vi "Host - Initialise and clone (SubVI).vi"(7 "Pilot":bool, 8 "error in":errorcluster, 10 "Tab Reference":refnum<vi>) -> (0 "error out":errorcluster, 2 "Control names":string[](array[string]), 3 "Data Cluster":T2={"VI References"=[], "Addresses"=[], "Pilot"=FALSE, "DO Data"=[], "Access Restricted?"=FALSE, "Pilot Control References"=[], "CoPilot Control References"=[], "cRIO Config"=[], "datalog Q"=refnum, "PS_P"={"AI"=[], "DI"=[], "DO"=[], "Serial"=[], "CPU"={"Total Load"=[], "Interrupt Load"=[], "Total Physical"=0.0, "Free Physical"=0.0, "Primary Disk Capacity"=0.0, "Primary Disk Free"=0.0}, "Stop"=FALSE, "DO Channel"=[]}, "PS_S"={"AI"=[], "DI"=[], "DO"=[], "Serial"=[], "CPU"={"Total Load"=[], "Interrupt Load"=[], "Total Physical"=0.0, "Free Physical"=0.0, "Primary Disk Capacity"=0.0, "Primary Disk Free"=0.0}, "Stop"=FALSE, "DO Channel"=[]}, "IDE_P"={"AI"=[], "DI"=[], "DO"=[], "Serial"=[], "CPU"={"Total Load"=[], "Interrupt Load"=[], "Total Physical"=0.0, "Free Physical"=0.0, "Primary Disk Capacity"=0.0, "Primary Disk Free"=0.0}, "Stop"=FALSE, "DO Channel"=[]}, "IDE_S"={"AI"=[], "DI"=[], "DO"=[], "Serial"=[], "CPU"={"Total Load"=[], "Interrupt Load"=[], "Total Physical"=0.0, "Free Physical"=0.0, "Primary Disk Capacity"=0.0, "Primary Disk Free"=0.0}, "Stop"=FALSE, "DO Channel"=[]}, "PDE_P"={"AI"=[], "DI"=[], "DO"=[], "Serial"=[], "CPU"={"Total Load"=[], "Interrupt Load"=[], "Total Physical"=0.0, "Free Physical"=0.0, "Primary Disk Capacity"=0.0, "Primary Disk Free"=0.0}, "Stop"=FALSE, "DO Channel"=[]}, "PDE_S"={"AI"=[], "DI"=[], "DO"=[], "Serial"=[], "CPU"={"Total Load"=[], "Interrupt Load"=[], "Total Physical"=0.0, "Free Physical"=0.0, "Primary Disk Capacity"=0.0, "Primary Disk Free"=0.0}, "Stop"=FALSE, "DO Channel"=[]}, "GUI References"={"Control Names"=[], "Control References"=[]}, "GUI Data"=[], "TCP - Serial"=[], "TCP-Serial Q"=refnum, "TCP Serial Ref"=[], "Data Sets"=[], "Last Data"=[], "Alarm Data"=[], "DI Data"=[], "Ack Data"=[], "Buzzer Data"=[], "Pilot DO"=[], "Co-Pilot DO"=[], "System Down?"=FALSE, "Log Data"=[], "Update Array"=[], "MCC Data Log"=[], "MCC Data Not"=refnum, "Thruster control"=[refnum, refnum, refnum, refnum, refnum, refnum, refnum, refnum, refnum], "waga notifier out"=refnum, "Wago  log"=[], "Thruster Cont"=[0.0, 0.0, 0.0, 0.0, 0.0, 0.0, 0.0, 0.0, 0.0], "Cam Cont"=[FALSE, FALSE, FALSE, FALSE, FALSE, TRUE], "PDE_P TH Cont"={"COM 10"=0.0, "COM 11"=0.0, "COM 12"=0.0, "COM 13"=0.0}, "PDE_S TH Cont"={"COM 10"=0.0, "COM 11"=0.0, "COM 12"=0.0, "COM 13"=0.0}} {"cRIO Config"."AI"."Interface Data"."Timing"."sample mode" items=["Finite Samples"=10178, "Continuous Samples"=10123, "Hardware Timed Single Point"=12522]; "cRIO Config"."Async"."Interface Data"."Data"."Minor Frame Count" min=5 max=8 step=1})   [LabVIEW 2021]
uses:
  Analog Output/Controls/AO Channel Configuration Cluster.ctl
  Analog Output/Controls/AO Timing Cluster.ctl
  Analog Output/Controls/AO Interface Data Cluster.ctl
  Analog Output/Controls/AO JSON Data Cluster.ctl
  Digital Output/SubVIs/Digital Dynamic Cluster.ctl
  Digital Output/Controls/DIO Interface Data.ctl
  Digital Output/Controls/DIO Configuration cluster.ctl
  Async Serial/Controls/Async Message Info Cluster.ctl
  Async Serial/Controls/Async Frame Info Cluster.ctl
  Async Serial/Controls/Async Serial Configuration Cluster.ctl
  Async Interface Data Cluster.ctl
  Async JSON Cluster.ctl
  Main Engine/Controls/Main Engine CPU Info.ctl
  Controls/Host Data Cluster.ctl
  Controls/Host - GUI Data Cluster.ctl
  Async Serial/Controls/Async Sensor Type.ctl
panel:
  out "Array":u32[](array[numeric])
  out "output array":refnum<vi>[](array[refnum])
  out "Names 3":string[](array[string])
  out "Names":string[](array[string])
  in  "Sensor Type":T1=enum."INS"
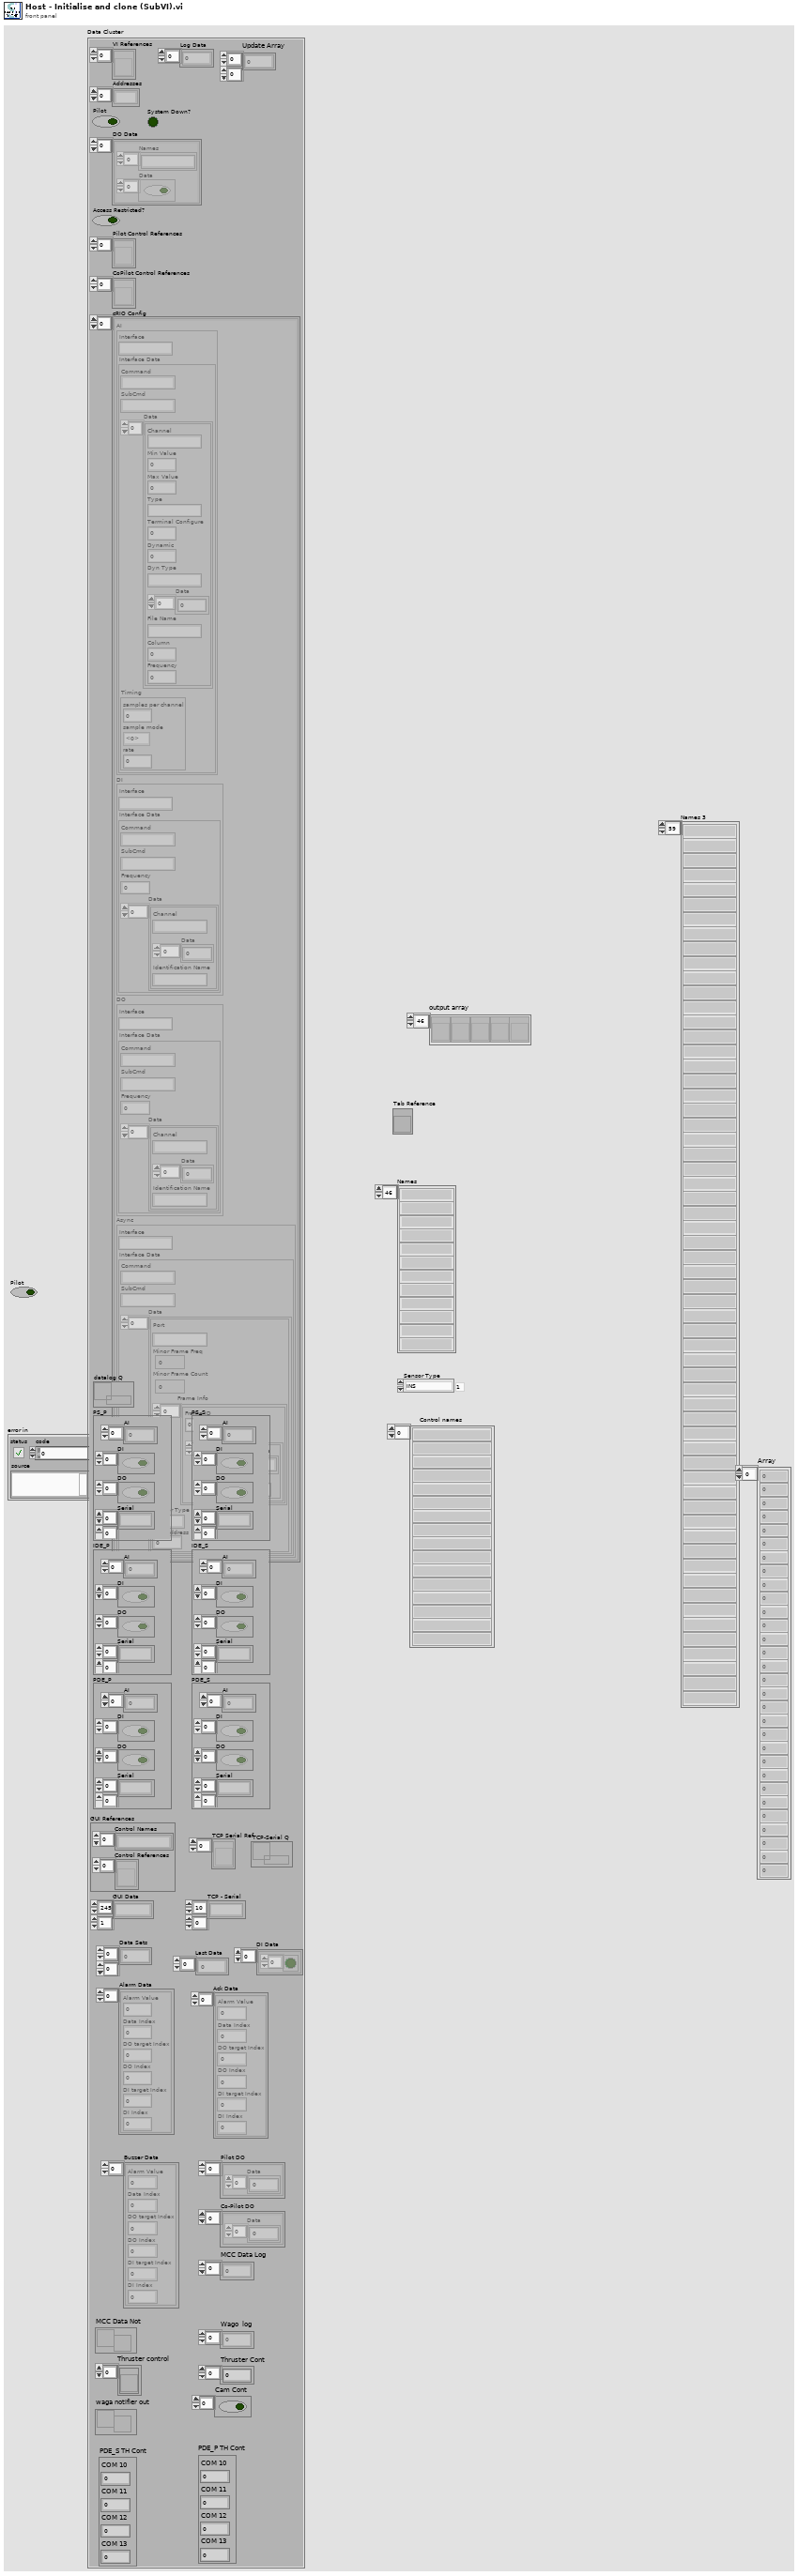
[diagram p1: front panel]
types:
  T1 = typedef "Async Sensor Type.ctl" = enum16{"Camera", "INS", "Pri BMS", "Aux BMS", "Depth Sensor", "Altimeter", "OIM", "Thruster", "Acoustic Modem", "LED"}
  T2 = typedef "Host - GUI Data Cluster.ctl" = cluster{"VI References":refnum<vi>[], "Addresses":string[], "Pilot":bool, "DO Data":cluster{"Names":string[], "Data":bool[]}[], "Access Restricted?":bool, "Pilot Control References":refnum<vi>[], "CoPilot Control References":refnum<vi>[], "cRIO Config":cluster{"AI":T3, "DI":T7, "DO":T7, "Async":T10}[], "datalog Q":refnum<queue>, "PS_P":T15, "PS_S":T15, "IDE_P":T15, "IDE_S":T15, "PDE_P":T15, "PDE_S":T15, "GUI References":cluster{"Control Names":string[], "Control References":refnum<vi>[]}, "GUI Data":string[][], "TCP - Serial":string[][], "TCP-Serial Q":refnum<queue>, "TCP Serial Ref":refnum<vi>[], "Data Sets":dbl[][], "Last Data":dbl[], "Alarm Data":cluster{"Alarm Value":dbl, "Data Index":i32, "DO target Index":i32, "DO Index":i32, "DI target Index":i32, "DI Index":i32}[], "DI Data":cluster{bool[]}[], "Ack Data":cluster{"Alarm Value":dbl, "Data Index":i32, "DO target Index":i32, "DO Index":i32, "DI target Index":i32, "DI Index":i32}[], "Buzzer Data":cluster{"Alarm Value":dbl, "Data Index":i32, "DO target Index":i32, "DO Index":i32, "DI target Index":i32, "DI Index":i32}[], "Pilot DO":cluster{"Data":i32[]}[], "Co-Pilot DO":cluster{"Data":i32[]}[], "System Down?":bool, "Log Data":dbl[], "Update Array":i32[][], "MCC Data Log":dbl[], "MCC Data Not":refnum<notifier>, "Thruster control":refnum<vi>[], "waga notifier out":refnum<notifier>, "Wago  log":sgl[], "Thruster Cont":dbl[], "Cam Cont":bool[], "PDE_P TH Cont":cluster{"COM 10":dbl, "COM 11":dbl, "COM 12":dbl, "COM 13":dbl}, "PDE_S TH Cont":cluster{"COM 10":dbl, "COM 11":dbl, "COM 12":dbl, "COM 13":dbl}}
  T3 = typedef "AO JSON Data Cluster.ctl" = cluster{"Interface":string, "Interface Data":T4}
  T4 = typedef "AO Interface Data Cluster.ctl" = cluster{"Command":string, "SubCmd":string, "Data":T5[], "Timing":T6}
  T5 = typedef "AO Channel Configuration Cluster.ctl" = cluster{"Channel":string, "Min Value":dbl, "Max Value":dbl, "Type":string, "Terminal Configure":u16, "Dynamic":u8, "Dyn Type":string, "Data":dbl[], "File Name":string, "Column":i32, "Frequency":dbl}
  T6 = typedef "AO Timing Cluster.ctl" = cluster{"samples per channel":i32, "sample mode":i32, "rate":dbl}
  T7 = typedef "DIO Configuration cluster.ctl" = cluster{"Interface":string, "Interface Data":T8}
  T8 = typedef "DIO Interface Data.ctl" = cluster{"Command":string, "SubCmd":string, "Frequency":u16, "Data":T9[]}
  T9 = typedef "Digital Dynamic Cluster.ctl" = cluster{"Channel":string, "Data":u8[], "Identification Name":string}
  T10 = typedef "Async JSON Cluster.ctl" = cluster{"Interface":string, "Interface Data":T11}
  T11 = typedef "Async Interface Data Cluster.ctl" = cluster{"Command":string, "SubCmd":string, "Data":T12[]}
  T12 = typedef "Async Serial Configuration Cluster.ctl" = cluster{"Port":string, "Minor Frame Freq":u16, "Minor Frame Count":u16, "Frame Info":T13[], "Sensor Type":u16, "OIM Address":u16}
  T13 = typedef "Async Frame Info Cluster.ctl" = cluster{"Frame ID":u16, "Message Info":T14[]}
  T14 = typedef "Async Message Info Cluster.ctl" = cluster{"Message":u8[], "Message Name":string}
  T15 = typedef "Host Data Cluster.ctl" = cluster{"AI":dbl[], "DI":bool[], "DO":bool[], "Serial":string[][], "CPU":T16, "Stop":bool, "DO Channel":string[]}
  T16 = typedef "Main Engine CPU Info.ctl" = cluster{"Total Load":u32[], "Interrupt Load":u32[], "Total Physical":dbl, "Free Physical":dbl, "Primary Disk Capacity":dbl, "Primary Disk Free":dbl}
  T17 = cluster{"AI":T3, "DI":T7, "DO":T7, "Async":T10}[]
  T18 = cluster{"Alarm Value":dbl, "Data Index":i32, "DO target Index":i32, "DO Index":i32, "DI target Index":i32, "DI Index":i32}[]
diagram:
  (unwired) string[][] [["IDE_P Voltage (V)", "IDE_P/AI/0", "3", "20", "PS_S/DO/0", "PS_S/DI/0", "0", "40", "25"], ["IDE_P_Voltage_2", "IDE_P/AI/1", "", "", "", "", "1", "-1", "-1"], ["IDE_P_Temp", "IDE_P/AI/2", "", "", "", "", "2", "-1", "27"], ["IDE_P Current (A)", "IDE_P/AI/3", ".05", "", "", "", "3", "41", "26"], ["IDE_P_Current_2", "IDE_P/AI/4", "", "", "", "", "4", "-1", "-1"], ["IDE_P WIS 1", "IDE_P/AI/5", "", "", "", "", "6", "-1", "-1"], ["IDE_P WIS 2", "IDE_P/AI/6", "", "", "", "", "7", "-1", "-1"], ["IDE_S Voltage (V)", "IDE_S/AI/0", "3", "", "", "", "8", "28", "20"], ["IDE_S_Voltage_2", "IDE_S/AI/1", "", "", "", "", "9", "-1", "-1"], ["IDE_S_Temp", "IDE_S/AI/2", "", "", "", "", "10", "-1", "22"], ["IDE_S Current (A)", "IDE_S/AI/3", "5", "", "", "", "11", "29", "21"], ["IDE_S_Current_2", "IDE_S/AI/4", "", "", "", "", "12", "-1", "-1"], ["IDE_S WIS 1", "IDE_S/AI/5", "", "", "", "", "14", "-1", "-1"], ["IDE_S WIS 2", "IDE_S/AI/6", "", "", "", "", "15", "-1", "-1"], ["PDE_P Voltage (V)", "PDE_P/AI/0", "16", "", "", "", "16", "38", "35"], ["PDE_P Current (A)", "PDE_P/AI/1", "30", "", "", "", "17", "39", "36"], ["PDE_P 24 Voltage1 (V)", "PDE_P/AI/2", "", "", "", "", "18", "-1", ""], ["PDE_P 24Current (A)", "PDE_P/AI/3", "", "", "", "", "19", "-1", ""], ["PDE_P 24 Voltage2 (V)", "PDE_P/AI/4", "", "", "", "", "20", "-1", ""], ["T1 Current", "PDE_P/AI/5", "7.5", "", "", "", "21", "-1", ""], ["T3 Current", "PDE_P/AI/6", "7.5", "", "", "", "22", "-1", ""], ["T5 Current", "PDE_P/AI/7", "7.5", "", "", "", "23", "-1", ""], ["T7 Current", "PDE_P/AI/8", "7.5", "", "", "", "24", "-1", ""], ["PDE_P BATS CUR", "PDE_P/AI/9", "", "", "", "", "25", "-1", ""], ["", "PDE_P/AI/10", "", "", "", "", "-1", "-1", ""], ["PDE_P Temp (degC)", "PDE_P/AI/12", "", "", "", "", "28", "-1", "37"], ["PDE_S Voltage (V)", "PDE_S/AI/0", "20", "", "", "", "29", "26", "30"], ["PDE_S Current (A)", "PDE_S/AI/1", "30", "", "", "", "30", "27", "31"], ["PDE_S24VOL1", "PDE_S/AI/2", "", "", "", "", "31", "-1", ""], ["PDE_S24V CUR", "PDE_S/AI/3", "", "", "", "", "32", "-1", ""], ["PDE_S24VOL2", "PDE_S/AI/4", "", "", "", "", "33", "-1", ""], ["T2 Current", "PDE_S/AI/5", "7.5", "", "", "", "34", "-1", ""], ["T4 Current", "PDE_S/AI/6", "7.5", "", "", "", "35", "-1", ""], ["T6 Current", "PDE_S/AI/7", "7.5", "", "", "", "36", "-1", ""], ["T8 Current", "PDE_S/AI/8", "7.5", "", "", "", "37", "-1", ""], ["PDE_S BATS CUR", "PDE_S/AI/9", "", "", "", "", "38", "-1", ""], ["LS01", "PDE_S/AI/10", "", "", "", "", "-1", "-1", ""], ["PDE_S_Temp", "PDE_S/AI/11", "", "", "", "", "41", "-1", "32"], ["4K camera P", "IDE_P/DO/0", "", "", "", "", "-1", "-1", ""], ["HD Camera P1", "IDE_P/DO/1", "", "", "", "", "-1", "-1", ""], ["HD Camera P2", "IDE_P/DO/2", "", "", "", "", "-1", "-1", ""], ["HD Camera P3", "IDE_P/DO/3", "", "", "", "", "-1", "-1", ""], ["SD_Camera_P4", "IDE_P/DO/4", "", "", "", "", "-1", "-1", ""], ["Pan and Tilt P1", "IDE_P/DO/5", "", "", "", "", "-1", "-1", ""], ["Laser Light 2", "IDE_P/DO/6", "", "", "", "", "-1", "-1", ""], ["LED Light P2", "IDE_P/DO/7", "", "", "", "", "-1", "-1", ""], ["LED Light P3", "IDE_P/DO/8", "", "", "", "", "-1", "-1", ""], ["LED Light P4", "IDE_P/DO/9", "", "", "", "", "-1", "-1", ""], ["Pan and Tilt P2", "IDE_P/DO/10", "", "", "", "", "-1", "-1", ""], ["Laser Light 1", "IDE_P/DO/11", "", "", "", "", "-1", "-1", ""], ["Depth Sensor Pri", "IDE_P/DO/12", "", "", "", "", "-1", "-1", ""], ["INS-DVL", "IDE_P/DO/13", "", "", "", "", "-1", "-1", ""], ["Multibeam Sonar", "IDE_P/DO/39", "", "", "", "", "-1", "-1", ""], ["SVP, Turbidity, pH", "IDE_P/DO/33", "", "", "", "", "-1", "-1", ""], ["CO2 Sensor", "IDE_P/DO/34", "", "", "", "", "-1", "-1", ""], ["Trim System", "IDE_P/DO/35", "", "", "", "", "-1", "-1", ""], ["Methane_Sensor", "IDE_P/DO/36", "", "", "", "", "-1", "-1", ""], ["VBS", "IDE_P/DO/37", "", "", "", "", "-1", "-1", ""], ["MBS", "IDE_P/DO/39", "", "", "", "", "-1", "-1", ""], ["4K camera S", "IDE_S/DO/0", "", "", "", "", "-1", "-1", ""], ["HD Camera S1", "IDE_S/DO/1", "", "", "", "", "-1", "-1", ""], ["HD Camera S2", "IDE_S/DO/2", "", "", "", "", "-1", "-1", ""], ["HD Camera S3", "IDE_S/DO/3", "", "", "", "", "-1", "-1", ""], ["SD Camera S4", "IDE_S/DO/4", "", "", "", "", "-1", "-1", ""], ["Pan and Tilt S", "IDE_S/DO/5", "", "", "", "", "-1", "-1", ""], ["Laser Light 3", "IDE_S/DO/6", "", "", "", "", "-1", "-1", ""], ["Laser Light 4", "IDE_S/DO/7", "", "", "", "", "-1", "-1", ""], ["LED Light S2", "IDE_S/DO/8", "", "", "", "", "-1", "-1", ""], ["LED Light S3", "IDE_S/DO/9", "", "", "", "", "-1", "-1", ""], ["LED Light S4", "IDE_S/DO/10", "", "", "", "", "-1", "-1", ""], ["Imaging Sonar", "IDE_S/DO/32", "", "", "", "", "-1", "-1", ""], ["Altimeter", "IDE_S/DO/33", "", "", "", "", "-1", "-1", ""], ["Subbottom Profiler", "IDE_S/DO/34", "", "", "", "", "-1", "-1", ""], ["Magnetometer", "IDE_S/DO/35", "", "", "", "", "-1", "-1", ""], ["Conduct & Temp", "IDE_S/DO/36", "", "", "", "", "-1", "-1", ""], ["Dissolved Oxygen", "IDE_S/DO/37", "", "", "", "", "86", "-1", ""], ["Plume Detector ", "IDE_S/DO/38", "", "", "", "", "-1", "-1", ""], ["Heat Probe Sensor", "IDE_S/DO/39", "", "", "", "", "-1", "-1", ""], ["Thrusters_T1", "", "", "", "", "", "-1", "-1", ""], ["Thrusters _T3", "", "", "", "", "", "-1", "-1", ""], ["Thrusters _T5", "", "", "", "", "", "-1", "-1", ""], ["Thrusters _T7", "", "", "", "", "", "-1", "-1", ""], ["T1Power", "PDE_P/DO/4", "", "", "", "", "-1", "-1", ""], ["T3Power", "PDE_P/DO/5", "", "", "", "", "-1", "-1", ""], ["T5Power", "PDE_P/DO/6", "", "", "", "", "-1", "-1", ""], ["T7Power", "PDE_P/DO/7", "", "", "", "", "-1", "-1", ""], ["BATS_P", "PDE_P/DO/8", "", "", "", "", "-1", "-1", ""], ["OIM RESET _P1", "PDE_P/DO/9", "", "", "", "", "-1", "-1", ""], ["OIM RESET_P2", "PDE_P/DO/10", "", "", "", "", "-1", "-1", ""], ["148 V LED P1", "PDE_P/DO/11", "", "", "", "", "-1", "-1", ""], ["148 V LED P2", "PDE_P/DO/12", "", "", "", "", "-1", "-1", ""], ["148 V LED P3", "PDE_P/DO/13", "", "", "", "", "-1", "-1", ""], ["148 V LED P4", "PDE_P/DO/14", "", "", "", "", "-1", "-1", ""], ["T2-Signal", "PDE_S/DO/0", "", "", "", "", "-1", "-1", ""], ["T4-Signal", "PDE_S/DO/1", "", "", "", "", "-1", "-1", ""], ["T6-Signal", "PDE_S/DO/2", "", "", "", "", "-1", "-1", ""], ["T8-Signal", "PDE_S/DO/3", "", "", "", "", "-1", "-1", ""], ["T2Power", "PDE_S/DO/4", "", "", "", "", "-1", "-1", ""], ["T4Power", "PDE_S/DO/5", "", "", "", "", "-1", "-1", ""], ["T6Power", "PDE_S/DO/6", "", "", "", "", "-1", "-1", ""], ["T8Power", "PDE_S/DO/7", "", "", "", "", "-1", "-1", ""], ["BATS_S", "PDE_S/DO/8", "", "", "", "", "-1", "-1", ""], ["OIM RESET _S1", "PDE_S/DO/9", "", "", "", "", "-1", "-1", ""], ["OIM RESET_S2", "PDE_S/DO/10", "", "", "", "", "-1", "-1", ""], ["148 V LED S1", "PDE_S/DO/11", "", "", "", "", "-1", "-1", ""], ["148 V LED S2", "PDE_S/DO/12", "", "", "", "", "-1", "-1", ""], ["148 V LED S3", "PDE_S/DO/13", "", "", "", "", "-1", "-1", ""], ["148 V LED S4", "PDE_S/DO/14", "", "", "", "", "-1", "-1", ""], ["T1-Signal", "PDE_P/DO/0", "", "", "", "", "-1", "-1", ""], ["T3-Signal", "PDE_P/DO/1", "", "", "", "", "-1", "-1", ""], ["T5-Signal", "PDE_P/DO/2", "", "", "", "", "-1", "-1", ""], ["T7-Signal", "PDE_P/DO/3", "", "", "", "", "-1", "-1", ""], ["Heading", "IDE_P/com1/1", "", "", "", "", "64", "-1", ""], ["Current (A)_P", "TCP/4004/1", "", "", "", "", "-1", "-1", ""], ["AUX_P Volt (V)", "TCP/4004/2", "", "", "", "", "-1", "-1", ""], ["AUX_P SOC (%)", "TCP/4004/3", "", "", "", "", "-1", "-1", ""], ["Roll", "IDE_P/com1/2", "", "", "", "", "62", "-1", ""], ["Pitch", "IDE_P/com1/3", "", "", "", "", "63", "-1", ""], ["Latitude", "IDE_P/com1/4", "", "", "", "", "65", "-1", ""], ["Longitude", "IDE_P/com1/5", "", "", "", "", "66", "-1", ""], ["Depth", "TCP/4003/1", "", "", "", "", "71", "-1", ""], ["Lateral\nSpeed", "IDE_P/com1/7", "", "", "", "", "68", "6", ""], ["Vertical    Speed", "IDE_P/com1/8", "", "", "", "", "69", "7", ""], ["Forward\nSpeed", "IDE_P/com1/9", "", "", "", "", "70", "8", ""], ["T2 Voltage", "PDE_S/com10/2", "", "", "", "", "139", "-1", ""], ["T2 Temp", "PDE_S/com10/6", "", "", "", "", "141", "-1", ""], ["T2 Speed", "PDE_S/com10/10", "", "", "", "", "138", "-1", ""], ["T4 Voltage", "PDE_S/com11/2", "", "", "", "", "143", "-1", ""], ["T4 Temp", "PDE_S/com11/6", "", "", "", "", "145", "-1", ""], ["T4 Speed", "PDE_S/com11/10", "", "", "", "", "143", "-1", ""], ["T6 Voltage", "PDE_S/com12/2", "", "", "", "", "147", "-1", ""], ["T6 Temp", "PDE_S/com12/6", "", "", "", "", "149", "-1", ""], ["T6 Speed", "PDE_S/com12/10", "", "", "", "", "146", "-1", ""], ["T8 Voltage", "PDE_S/com13/2", "", "", "", "", "151", "-1", ""], ["T8 Temp", "PDE_S/com13/6", "", "", "", "", "153", "-1", ""], ["T8 Speed", "PDE_S/com13/10", "", "", "", "", "150", "-1", ""], ["AUX_P Current (A)", "TCP/4002/4", "", "", "", "", "43", "35", ""], ["AUX_P Volt (V)", "TCP/4002/11", "", "", "", "", "42", "36", ""], ["AUX_P SOC (%)", "TCP/4002/10", "", "", "", "", "45", "37", ""], ["MB_P Volt (V)", "TCP/4007/2", "", "", "", "", "52", "32", ""], ["MP_P Current (A)", "TCP/4007/1", "", "", "", "", "53", "33", ""], ["MB_P SOC (%)", "TCP/4007/3", "", "", "", "", "55", "34", ""], ["MB_P Temp (deg C)", "TCP/4007/5", "", "", "", "", "56", "-1", ""], ["T1 Voltage", "PDE_P/com10/2", "", "", "", "", "123", "-1", ""], ["T1 Temp", "PDE_P/com10/6", "", "", "", "", "125", "-1", ""], ["T1 Speed", "PDE_P/com10/10", "", "", "", "", "122", "-1", ""], ["T3 Voltage", "PDE_P/com11/2", "", "", "", "", "127", "-1", ""], ["T3  Temp", "PDE_P/com11/6", "", "", "", "", "129", "-1", ""], ["T3 Speed", "PDE_P/com11/10", "", "", "", "", "126", "-1", ""], ["T5 Voltage", "PDE_P/com12/2", "", "", "", "", "131", "-1", ""], ["T5 Temp", "PDE_P/com12/6", "", "", "", "", "133", "-1", ""], ["T5 Speed", "PDE_P/com12/10", "", "", "", "", "130", "-1", ""], ["T7 Voltage", "PDE_P/com13/2", "", "", "", "", "135", "-1", ""], ["T7 Temp", "PDE_P/com13/6", "", "", "", "", "137", "-1", ""], ["T7 Speed", "PDE_P/com13/10", "", "", "", "", "134", "-1", ""], ["BAT CUR", "TCP/4007/1", "", "", "", "", "-1", "-1", ""], ["BAT VOL", "TCP/4007/2", "", "", "", "", "-1", "-1", ""], ["BAT SOC", "TCP/4007/3", "", "", "", "", "-1", "-1", ""], ["BAT TEMP", "TCP/4007/5", "", "", "", "", "-1", "-1", ""], ["Current_1", "TCP/4007/22", "", "", "", "", "162", "-1", ""], ["Voltage_1", "TCP/4007/23", "", "", "", "", "163", "-1", ""], ["ID Cell Max_1", "TCP/4007/24", "", "", "", "", "164", "-1", ""], ["Max Temp_1", "TCP/4007/25", "", "", "", "", "165", "-1", ""], ["ID Cell Min _1 ", "TCP/4007/26", "", "", "", "", "166", "-1", ""], ["Min Temp_1", "TCP/4007/27", "", "", "", "", "167", "-1", ""], ["Temp_1", "TCP/4007/28", "", "", "", "", "168", "-1", ""], ["SOC_1", "TCP/4007/29", "", "", "", "", "169", "-1", ""], ["SOH_1", "TCP/4007/30", "", "", "", "", "170", "-1", ""], ["Current_2", "TCP/4007/37", "", "", "", "", "171", "-1", ""], ["Voltage_2", "TCP/4007/38", "", "", "", "", "172", "-1", ""], ["ID Cell Max_2", "TCP/4007/39", "", "", "", "", "173", "-1", ""], ["Max Temp_2", "TCP/4007/40", "", "", "", "", "174", "-1", ""], ["ID Cell Min _2", "TCP/4007/41", "", "", "", "", "175", "-1", ""], ["Min Temp_2", "TCP/4007/42", "", "", "", "", "176", "-1", ""], ["Temp_2", "TCP/4007/43", "", "", "", "", "177", "-1", ""], ["SOC_2", "TCP/4007/44", "", "", "", "", "178", "-1", ""], ["SOH_2", "TCP/4007/45", "", "", "", "", "179", "-1", ""], ["Current_3", "TCP/4007/52", "", "", "", "", "180", "-1", ""], ["Voltage_3", "TCP/4007/53", "", "", "", "", "181", "-1", ""], ["ID Cell Max_3", "TCP/4007/54", "", "", "", "", "182", "-1", ""], ["Max Temp_3", "TCP/4007/55", "", "", "", "", "183", "-1", ""], ["ID Cell Min _3", "TCP/4007/56", "", "", "", "", "184", "-1", ""], ["Min Temp_3", "TCP/4007/57", "", "", "", "", "185", "-1", ""], ["Temp_3", "TCP/4007/58", "", "", "", "", "186", "-1", ""], ["SOC_3", "TCP/4007/59", "", "", "", "", "187", "-1", ""], ["SOH_3", "TCP/4007/60", "", "", "", "", "188", "-1", ""], ["Current_4", "TCP/4007/67", "", "", "", "", "189", "-1", ""], ["Voltage_4", "TCP/4007/68", "", "", "", "", "190", "-1", ""], ["ID Cell Max_4", "TCP/4007/69", "", "", "", "", "191", "-1", ""], ["Max Temp_4", "TCP/4007/70", "", "", "", "", "192", "-1", ""], ["ID Cell Min _4", "TCP/4007/71", "", "", "", "", "193", "-1", ""], ["Min Temp_4", "TCP/4007/72", "", "", "", "", "194", "-1", ""], ["Temp_4", "TCP/4007/73", "", "", "", "", "195", "-1", ""], ["SOC_4", "TCP/4007/74", "", "", "", "", "196", "-1", ""], ["SOH_4", "TCP/4007/75", "", "", "", "", "197", "-1", ""], ["Current_5", "TCP/4007/82", "", "", "", "", "198", "-1", ""], ["Voltage_5", "TCP/4007/83", "", "", "", "", "199", "-1", ""], ["ID Cell Max_5", "TCP/4007/84", "", "", "", "", "200", "-1", ""], ["Max Temp_5", "TCP/4007/85", "", "", "", "", "201", "-1", ""], ["ID Cell Min _5", "TCP/4007/86", "", "", "", "", "202", "-1", ""], ["Min Temp_5", "TCP/4007/87", "", "", "", "", "203", "-1", ""], ["Temp_5", "TCP/4007/88", "", "", "", "", "204", "-1", ""], ["SOC_5", "TCP/4007/89", "", "", "", "", "205", "-1", ""], ["SOH_5", "TCP/4007/90", "", "", "", "", "206", "-1", ""], ["Altitude", "TCP/4009/1", "", "", "", "", "67", "5", ""], ["S_Heading", "TCP/8110/1", "", "", "", "", "74", "0", ""], ["S_Roll", "TCP/8110/2", "", "", "", "", "72", "1", ""], ["S_Pitch", "TCP/8110/3", "", "", "", "", "73", "2", ""], ["S_Latitude", "TCP/8110/4", "", "", "", "", "75", "3", ""], ["S_Longitude", "TCP/8110/5", "", "", "", "", "76", "4", ""], ["S_Depth", "TCP/4010/1", "", "", "", "", "77", "9", ""], ["T1 ctrl", " PDE_P/com10/9", "", "", "", "", "154", "-1", ""], ["T3 ctrl", " PDE_P/com11/9", "", "", "", "", "155", "-1", ""], ["T5 ctrl", " PDE_P/com12/9", "", "", "", "", "156", "-1", ""], ["T7 ctrl ", " PDE_P/com13/9", "", "", "", "", "157", "-1", ""], ["T2 ctrl ", " PDE_S/com10/9", "", "", "", "", "158", "-1", ""], ["T4 ctrl", " PDE_S/com11/9", "", "", "", "", "159", "-1", ""], ["T6 ctrl", " PDE_S/com12/9", "", "", "", "", "160", "-1", ""], ["T8 ctrl", " PDE_S/com13/9", "", "", "", "", "161", "-1", ""], ["CO2_s ", "", "", "", "", "", "91", "10", ""], ["Oxygen_S", "", "", "", "", "", "92", "11", ""], ["Presssure in mbar_S", "", "", "", "", "", "93", "12", ""], ["Temp in Deg C_S", "", "", "", "", "", "94", "13", ""], ["Humidity_S in %", "", "", "", "", "", "95", "14", ""], ["CO2_P ", "", "", "", "", "", "101", "15", ""], ["Oxygen_P", "", "", "", "", "", "102", "16", ""], ["Presssure in mbar_P", "", "", "", "", "", "103", "17", ""], ["Temp in Deg C_P", "", "", "", "", "", "104", "18", ""], ["Humidity_P in %", "", "", "", "", "", "105", "19", ""], ["MB_S Volt (V)", "", "", "", "", "", "57", "20", ""], ["MB_S Current (A)", "", "", "", "", "", "58", "21", ""], ["MB_S SOC (%)", "", "", "", "", "", "60", "22", ""], ["AUX_S Volt (V)", "", "", "", "", "", "47", "23", ""], ["AUX_S Current (A)", "", "", "", "", "", "48", "24", ""], ["AUX_S SOC (%)", "", "", "", "", "", "50", "25", ""], ["PDE_S IR (Kohm)", "", "", "", "", "", "-1", "30", ""], ["IDE_S IR  (Kohm)", "", "", "", "", "", "-1", "31", ""], ["PDE_P IR (Kohm)", "", "", "", "", "", "-1", "42", ""], ["IDE_P IR (kohm)", "", "", "", "", "", "-1", "43", ""], ["S_ALGSTS_M", "TCP/8110/16", "", "", "", "", "-1", "-1", ""], ["S_ALGSTS_L", "TCP/8110/17", "", "", "", "", "-1", "-1", ""], ["S_STATUS_M", "TCP/8110/18", "", "", "", "", "-1", "-1", ""], ["S_STATUS_L", "TCP/8110/19", "", "", "", "", "-1", "-1", ""], ["S_HTSTATUS", "TCP/8110/20", "", "", "", "", "-1", "-1", ""], ["Dissolved O2", "IDE_S/DO/12", "", "", "", "", "-1", "-1", ""]]
  (unwired) string[] ["", "", "", "", "192.168.81.150", ""]
  (unwired) string[][] [["IDE_P Voltage (V)", "IDE_P/AI/0", "3", "20", "PS_S/DO/0", "PS_S/DI/0", "0"], ["IDE_P_Voltage_2", "IDE_P/AI/1", "", "", "", "", "1"], ["IDE_P_Temp", "IDE_P/AI/2", "", "", "", "", "2"], ["IDE_P Current (A)", "IDE_P/AI/3", ".05", "", "", "", "3"], ["IDE_P_Current_2", "IDE_P/AI/4", "", "", "", "", "4"], ["", "IDE_P/AI/5", "", "", "", "", "-1"], ["", "IDE_P/AI/6", "", "", "", "", "-1"], ["IDE_S Voltage (V)", "IDE_S/AI/0", "3", "", "", "", "5"], ["IDE_S_Voltage_2", "IDE_S/AI/1", "", "", "", "", "6"], ["IDE_S_Temp", "IDE_S/AI/2", "", "", "", "", "7"], ["IDE_S Current (A)", "IDE_S/AI/3", "5", "", "", "", "8"], ["IDE_S_Current_2", "IDE_S/AI/4", "", "", "", "", "9"], ["", "IDE_S/AI/5", "", "", "", "", "-1"], ["", "IDE_S/AI/6", "", "", "", "", "-1"], ["PDE_P Voltage (V)", "PDE_P/AI/0", "20", "", "", "", "10"], ["PDE_P Current (A)", "PDE_P/AI/1", "30", "", "", "", "11"], ["", "PDE_P/AI/2", "", "", "", "", "-1"], ["", "PDE_P/AI/3", "", "", "", "", "-1"], ["", "PDE_P/AI/4", "", "", "", "", "-1"], ["T1 Current", "PDE_P/AI/5", "7.5", "", "", "", "-1"], ["T3 Current", "PDE_P/AI/6", "7.5", "", "", "", "-1"], ["T5 Current", "PDE_P/AI/7", "7.5", "", "", "", "-1"], ["T7 Current", "PDE_P/AI/8", "7.5", "", "", "", "-1"], ["", "PDE_P/AI/9", "", "", "", "", "-1"], ["", "PDE_P/AI/10", "", "", "", "", "-1"], ["PDE_P_Temp", "PDE_P/AI/11", "", "", "", "", "12"], ["PDE_S Voltage (V)", "PDE_S/AI/0", "20", "", "", "", "13"], ["PDE_S Current (A)", "PDE_S/AI/1", "30", "", "", "", "14"], ["", "PDE_S/AI/2", "", "", "", "", "-1"], ["", "PDE_S/AI/3", "", "", "", "", "-1"], ["", "PDE_S/AI/4", "", "", "", "", "-1"], ["T2 Current", "PDE_S/AI/5", "7.5", "", "", "", "-1"], ["T4 Current", "PDE_S/AI/6", "7.5", "", "", "", "-1"], ["T6 Current", "PDE_S/AI/7", "7.5", "", "", "", "-1"], ["T8 Current", "PDE_S/AI/8", "7.5", "", "", "", "-1"], ["", "PDE_S/AI/9", "", "", "", "", "-1"], ["", "PDE_S/AI/10", "", "", "", "", "-1"], ["PDE_S_Temp", "PDE_S/AI/11", "", "", "", "", "29"], ["4K camera P", "IDE_P/DO/0", "", "", "", "", "-1"], ["HD Camera P1", "IDE_P/DO/1", "", "", "", "", "-1"], ["HD Camera P2", "IDE_P/DO/2", "", "", "", "", "-1"], ["HD Camera P3", "IDE_P/DO/3", "", "", "", "", "-1"], ["SD_Camera_P4", "IDE_P/DO/4", "", "", "", "", ""], ["Pan and Tilt P1", "IDE_P/DO/5", "", "", "", "", ""], ["Laser Light 2", "IDE_P/DO/6", "", "", "", "", ""], ["LED Light P2", "IDE_P/DO/7", "", "", "", "", ""], ["LED Light P3", "IDE_P/DO/8", "", "", "", "", ""], ["LED Light P4", "IDE_P/DO/9", "", "", "", "", ""], ["Pan and Tilt P2", "IDE_P/DO/10", "", "", "", "", ""], ["Laser Light 1", "IDE_P/DO/11", "", "", "", "", ""], ["Depth Sensor Pri", "IDE_P/DO/12", "", "", "", "", ""], ["INS-DVL", "IDE_P/DO/13", "", "", "", "", ""], ["Multibeam Sonar", "IDE_P/DO/39", "", "", "", "", ""], ["SVP, Turbidity, pH", "IDE_P/DO/33", "", "", "", "", ""], ["CO2 Sensor", "IDE_P/DO/34", "", "", "", "", ""], ["Trim System", "IDE_P/DO/35", "", "", "", "", ""], ["Methane_Sensor", "IDE_P/DO/36", "", "", "", "", ""], ["VBS", "IDE_P/DO/37", "", "", "", "", ""], ["MBS", "IDE_P/DO/39", "", "", "", "", ""], ["4K camera S", "IDE_S/DO/0", "", "", "", "", ""], ["HD Camera S1", "IDE_S/DO/1", "", "", "", "", ""], ["HD Camera S2", "IDE_S/DO/2", "", "", "", "", ""], ["HD Camera S3", "IDE_S/DO/3", "", "", "", "", ""], ["SD Camera S4", "IDE_S/DO/4", "", "", "", "", ""], ["Pan and Tilt S", "IDE_S/DO/5", "", "", "", "", ""], ["Laser Light 3", "IDE_S/DO/6", "", "", "", "", ""], ["Laser Light 4", "IDE_S/DO/7", "", "", "", "", ""], ["LED Light S2", "IDE_S/DO/8", "", "", "", "", ""], ["LED Light S3", "IDE_S/DO/9", "", "", "", "", ""], ["LED Light S4", "IDE_S/DO/10", "", "", "", "", ""], ["Imaging Sonar", "IDE_S/DO/32", "", "", "", "", ""], ["Altimeter", "IDE_S/DO/33", "", "", "", "", ""], ["Subbottom Profiler", "IDE_S/DO/34", "", "", "", "", ""], ["Magnetometer", "IDE_S/DO/35", "", "", "", "", ""], ["Conduct & Temp", "IDE_S/DO/36", "", "", "", "", ""], ["Dissolved Oxygen", "IDE_S/DO/37", "", "", "", "", ""], ["Plume Detector ", "IDE_S/DO/38", "", "", "", "", ""], ["Heat Probe Sensor", "IDE_S/DO/39", "", "", "", "", ""], ["Thrusters_T1", "", "", "", "", "", ""], ["Thrusters _T3", "", "", "", "", "", ""], ["Thrusters _T5", "", "", "", "", "", ""], ["Thrusters _T7", "", "", "", "", "", ""], ["T1Power", "PDE_P/DO/4", "", "", "", "", ""], ["T3Power", "PDE_P/DO/5", "", "", "", "", ""], ["T5Power", "PDE_P/DO/6", "", "", "", "", ""], ["T7Power", "PDE_P/DO/7", "", "", "", "", ""], ["BATS_P", "PDE_P/DO/8", "", "", "", "", ""], ["OIM RESET _P1", "PDE_P/DO/9", "", "", "", "", ""], ["OIM RESET_P2", "PDE_P/DO/10", "", "", "", "", ""], ["148 V LED P1", "PDE_P/DO/11", "", "", "", "", ""], ["148 V LED P2", "PDE_P/DO/12", "", "", "", "", ""], ["148 V LED P3", "PDE_P/DO/13", "", "", "", "", ""], ["148 V LED P4", "PDE_P/DO/14", "", "", "", "", ""], ["T2-Signal", "PDE_S/DO/0", "", "", "", "", ""], ["T4-Signal", "PDE_S/DO/1", "", "", "", "", ""], ["T6-Signal", "PDE_S/DO/2", "", "", "", "", ""], ["T8-Signal", "PDE_S/DO/3", "", "", "", "", ""], ["T2Power", "PDE_S/DO/4", "", "", "", "", ""], ["T4Power", "PDE_S/DO/5", "", "", "", "", ""], ["T6Power", "PDE_S/DO/6", "", "", "", "", ""], ["T8Power", "PDE_S/DO/7", "", "", "", "", ""], ["BATS_S", "PDE_S/DO/8", "", "", "", "", ""], ["OIM RESET _S1", "PDE_S/DO/9", "", "", "", "", ""], ["OIM RESET_S2", "PDE_S/DO/10", "", "", "", "", ""], ["148 V LED S1", "PDE_S/DO/11", "", "", "", "", ""], ["148 V LED S2", "PDE_S/DO/12", "", "", "", "", ""], ["148 V LED S3", "PDE_S/DO/13", "", "", "", "", ""], ["148 V LED S4", "PDE_S/DO/14", "", "", "", "", ""], ["T1-Signal", "PDE_P/DO/0", "", "", "", "", ""], ["T3-Signal", "PDE_P/DO/1", "", "", "", "", ""], ["T5-Signal", "PDE_P/DO/2", "", "", "", "", ""], ["T7-Signal", "PDE_P/DO/3", "", "", "", "", ""], ["Heading", "IDE_P/com1/1", "", "", "", "", ""], ["Current (A)_P", "TCP/4004/1", "", "", "", "", ""], ["AUX_P Volt (V)", "TCP/4004/2", "", "", "", "", ""], ["AUX_P SOC (%)", "TCP/4004/3", "", "", "", "", ""], ["Roll", "IDE_P/com1/2", "", "", "", "", ""], ["Pitch", "IDE_P/com1/3", "", "", "", "", ""], ["Latitude", "IDE_P/com1/4", "", "", "", "", ""], ["Longitude", "IDE_P/com1/5", "", "", "", "", ""], ["Depth", "TCP/4003/1", "", "", "", "", ""], ["Lateral\nSpeed", "IDE_P/com1/7", "", "", "", "", ""], ["Vertical    Speed", "IDE_P/com1/8", "", "", "", "", ""], ["Forward\nSpeed", "IDE_P/com1/9", "", "", "", "", ""], ["T2 Voltage", "PDE_S/com10/2", "", "", "", "", ""], ["T2 Temp", "PDE_S/com10/6", "", "", "", "", ""], ["T2 Speed", "PDE_S/com10/10", "", "", "", "", ""], ["T4 Voltage", "PDE_S/com11/2", "", "", "", "", ""], ["T4 Temp", "PDE_S/com11/6", "", "", "", "", ""], ["T4 Speed", "PDE_S/com11/10", "", "", "", "", ""], ["T6 Voltage", "PDE_S/com12/2", "", "", "", "", ""], ["T6 Temp", "PDE_S/com12/6", "", "", "", "", ""], ["T6 Speed", "PDE_S/com12/10", "", "", "", "", ""], ["T8 Voltage", "PDE_S/com13/2", "", "", "", "", ""], ["T8 Temp", "PDE_S/com13/6", "", "", "", "", ""], ["T8 Speed", "PDE_S/com13/10", "", "", "", "", ""], ["Current (A)_P", "TCP/4002/4", "", "", "", "", ""], ["AUX_P Volt (V)", "TCP/4002/11", "", "", "", "", ""], ["AUX_P SOC (%)", "TCP/4002/10", "", "", "", "", ""], ["MB_P Volt (V)", "TCP/4007/2", "", "", "", "", ""], ["MP_P Current (A)", "TCP/4007/1", "", "", "", "", ""], ["MB_P SOC (%)", "TCP/4007/3", "", "", "", "", ""], ["MB_P Temp (deg C)", "TCP/4007/5", "", "", "", "", ""], ["T1 Voltage", "PDE_P/com10/2", "", "", "", "", ""], ["T1 Temp", "PDE_P/com10/6", "", "", "", "", ""], ["T1 Speed", "PDE_P/com10/10", "", "", "", "", ""], ["T3 Voltage", "PDE_P/com11/2", "", "", "", "", ""], ["T3  Temp", "PDE_P/com11/6", "", "", "", "", ""], ["T3 Speed", "PDE_P/com11/10", "", "", "", "", ""], ["T5 Voltage", "PDE_P/com12/2", "", "", "", "", ""], ["T5 Temp", "PDE_P/com12/6", "", "", "", "", ""], ["T5 Speed", "PDE_P/com12/10", "", "", "", "", ""], ["T7 Voltage", "PDE_P/com13/2", "", "", "", "", ""], ["T7 Temp", "PDE_P/com13/6", "", "", "", "", ""], ["T7 Speed", "PDE_P/com13/10", "", "", "", "", ""], ["BAT CUR", "TCP/4007/1", "", "", "", "", ""], ["BAT VOL", "TCP/4007/2", "", "", "", "", ""], ["BAT SOC", "TCP/4007/3", "", "", "", "", ""], ["BAT TEMP", "TCP/4007/5", "", "", "", "", ""], ["Current_1", "TCP/4007/22", "", "", "", "", ""], ["Voltage_1", "TCP/4007/23", "", "", "", "", ""], ["ID Cell Max_1", "TCP/4007/24", "", "", "", "", ""], ["Max Temp_1", "TCP/4007/25", "", "", "", "", ""], ["ID Cell Min _1 ", "TCP/4007/26", "", "", "", "", ""], ["Min Temp_1", "TCP/4007/27", "", "", "", "", ""], ["Temp_1", "TCP/4007/28", "", "", "", "", ""], ["SOC_1", "TCP/4007/29", "", "", "", "", ""], ["SOH_1", "TCP/4007/30", "", "", "", "", ""], ["Current_2", "TCP/4007/37", "", "", "", "", ""], ["Voltage_2", "TCP/4007/38", "", "", "", "", ""], ["ID Cell Max_2", "TCP/4007/39", "", "", "", "", ""], ["Max Temp_2", "TCP/4007/40", "", "", "", "", ""], ["ID Cell Min _2", "TCP/4007/41", "", "", "", "", ""], ["Min Temp_2", "TCP/4007/42", "", "", "", "", ""], ["Temp_2", "TCP/4007/43", "", "", "", "", ""], ["SOC_2", "TCP/4007/44", "", "", "", "", ""], ["SOH_2", "TCP/4007/45", "", "", "", "", ""], ["Current_3", "TCP/4007/52", "", "", "", "", ""], ["Voltage_3", "TCP/4007/53", "", "", "", "", ""], ["ID Cell Max_3", "TCP/4007/54", "", "", "", "", ""], ["Max Temp_3", "TCP/4007/55", "", "", "", "", ""], ["ID Cell Min _3", "TCP/4007/56", "", "", "", "", ""], ["Min Temp_3", "TCP/4007/57", "", "", "", "", ""], ["Temp_3", "TCP/4007/58", "", "", "", "", ""], ["SOC_3", "TCP/4007/59", "", "", "", "", ""], ["SOH_3", "TCP/4007/60", "", "", "", "", ""], ["Current_4", "TCP/4007/67", "", "", "", "", ""], ["Voltage_4", "TCP/4007/68", "", "", "", "", ""], ["ID Cell Max_4", "TCP/4007/69", "", "", "", "", ""], ["Max Temp_4", "TCP/4007/70", "", "", "", "", ""], ["ID Cell Min _4", "TCP/4007/71", "", "", "", "", ""], ["Min Temp_4", "TCP/4007/72", "", "", "", "", ""], ["Temp_4", "TCP/4007/73", "", "", "", "", ""], ["SOC_4", "TCP/4007/74", "", "", "", "", ""], ["SOH_4", "TCP/4007/75", "", "", "", "", ""], ["Current_5", "TCP/4007/82", "", "", "", "", ""], ["Voltage_5", "TCP/4007/83", "", "", "", "", ""], ["ID Cell Max_5", "TCP/4007/84", "", "", "", "", ""], ["Max Temp_5", "TCP/4007/85", "", "", "", "", ""], ["ID Cell Min _5", "TCP/4007/86", "", "", "", "", ""], ["Min Temp_5", "TCP/4007/87", "", "", "", "", ""], ["Temp_5", "TCP/4007/88", "", "", "", "", ""], ["SOC_5", "TCP/4007/89", "", "", "", "", ""], ["SOH_5", "TCP/4007/90", "", "", "", "", ""], ["Altitude", "TCP/4009/1", "", "", "", "", ""], ["S_Heading", "TCP/8110/1", "", "", "", "", ""], ["S_Roll", "TCP/8110/2", "", "", "", "", ""], ["S_Pitch", "TCP/8110/3", "", "", "", "", ""], ["S_Latitude", "TCP/8110/4", "", "", "", "", ""], ["S_Longitude", "TCP/8110/5", "", "", "", "", ""], ["S_Depth", "TCP/4010/1", "", "", "", "", ""]]
  w15 = sgl 0.0 ("element")
  w2 = string[] ["192.168.81.50", "192.168.81.100", "192.168.81.10", "192.168.81.170", "192.168.81.150", "192.168.81.120"]  # Source
  w1 = string[][] [["IDE_P Voltage (V)", "IDE_P/AI/0", "3", "20", "PS_S/DO/0", "PS_S/DI/0", "1", "40", "25"], ["IDE_P_Voltage_2", "IDE_P/AI/1", "", "", "", "", "2", "-1", "-1"], ["IDE_P_Temp", "IDE_P/AI/2", "", "", "", "", "3", "-1", "27"], ["IDE_P Current (A)", "IDE_P/AI/3", "5", "", "", "", "4", "41", "26"], ["IDE_P_Current_2", "IDE_P/AI/4", "", "", "", "", "5", "-1", "-1"], ["IDE_P WIS 1", "IDE_P/AI/5", "", "", "", "", "7", "-1", "-1"], ["IDE_P WIS 2", "IDE_P/AI/6", "", "", "", "", "8", "-1", "-1"], ["IDE_S Voltage (V)", "IDE_S/AI/0", "3", "", "", "", "268", "28", "20"], ["IDE_S_Voltage_2", "IDE_S/AI/1", "", "", "", "", "10", "-1", "-1"], ["IDE_S Temp (degC)", "IDE_S/AI/2", "10", "", "", "", "270", "-1", "22"], ["IDE_S Current (A)", "IDE_S/AI/4", "-5", "", "", "", "269", "29", "21"], ["IDE_S_Current_2", "IDE_S/AI/4", "", "", "", "", "13", "-1", "-1"], ["IDE_S WIS 1", "IDE_S/AI/5", "", "", "", "", "15", "-1", "-1"], ["IDE_S WIS 2", "IDE_S/AI/6", "", "", "", "", "17", "-1", "-1"], ["PDE_P Voltage (V)", "PDE_P/AI/0", "16", "", "", "", "18", "38", "35"], ["PDE_P Current (A)", "PDE_P/AI/1", "30", "", "", "", "-1", "39", "36"], ["PDE_P 24 Voltage1 (V)", "PDE_P/AI/2", "", "", "", "", "19", "-1", ""], ["PDE_P 24Current (A)", "PDE_P/AI/3", "", "", "", "", "20", "-1", ""], ["PDE_P 24 Voltage2 (V)", "PDE_P/AI/4", "", "", "", "", "21", "-1", ""], ["T1 Current", "PDE_P/AI/5", "7.5", "", "", "", "22", "-1", ""], ["T3 Current", "PDE_P/AI/6", "7.5", "", "", "", "23", "-1", ""], ["T5 Current", "PDE_P/AI/7", "7.5", "", "", "", "24", "-1", ""], ["T7 Current", "PDE_P/AI/8", "7.5", "", "", "", "25", "-1", ""], ["PDE_P BATS CUR", "PDE_P/AI/9", "", "", "", "", "26", "-1", ""], ["", "PDE_P/AI/10", "", "", "", "", "-1", "-1", ""], ["PDE_P Temp (degC)", "PDE_P/AI/12", "", "", "", "", "29", "-1", "37"], ["PDE_S Voltage (V)", "PDE_S/AI/0", "20", "", "", "", "264", "26", "30"], ["PDE_S Current (A)", "PDE_S/AI/1", "-30", "", "", "", "265", "27", "31"], ["PDE_S24VOL1", "PDE_S/AI/2", "", "", "", "", "32", "-1", ""], ["PDE_S24V CUR", "PDE_S/AI/3", "", "", "", "", "33", "-1", ""], ["PDE_S24VOL2", "PDE_S/AI/4", "", "", "", "", "34", "-1", ""], ["T2 Current", "PDE_S/com10/3", "", "", "", "", "273", "-1", ""], ["T4 Current", "PDE_S/com11/3", "", "", "", "", "279", "-1", ""], ["T6 Current", "PDE_S/com12/3", "", "", "", "", "285", "-1", ""], ["T8 Current", "PDE_S/com13/3", "", "", "", "", "291", "-1", ""], ["PDE_S BATS CUR", "PDE_S/AI/9", "", "", "", "", "39", "-1", ""], ["LS01", "PDE_S/AI/10", "", "", "", "", "40", "-1", ""], ["PDE_S Temp (degC)", "PDE_S/AI/12", "10", "", "", "", "266", "-1", "32"], ["4K camera P", "IDE_P/DO/0", "", "", "", "", "-1", "-1", ""], ["HD Camera P1", "IDE_P/DO/1", "", "", "", "", "-1", "-1", ""], ["HD Camera P2", "IDE_P/DO/2", "", "", "", "", "-1", "-1", ""], ["HD Camera P3", "IDE_P/DO/3", "", "", "", "", "-1", "-1", ""], ["SD_Camera_P4", "IDE_P/DO/4", "", "", "", "", "-1", "-1", ""], ["Pan and Tilt P1", "IDE_P/DO/5", "", "", "", "", "-1", "-1", ""], ["Laser Light 2", "IDE_P/DO/6", "", "", "", "", "-1", "-1", ""], ["LED Light P2", "IDE_P/DO/7", "", "", "", "", "-1", "-1", ""], ["LED Light P3", "IDE_P/DO/8", "", "", "", "", "-1", "-1", ""], ["LED Light P4", "IDE_P/DO/9", "", "", "", "", "-1", "-1", ""], ["Pan and Tilt P2", "IDE_P/DO/10", "", "", "", "", "-1", "-1", ""], ["Laser Light 1", "IDE_P/DO/11", "", "", "", "", "-1", "-1", ""], ["Depth Sensor Pri", "IDE_P/DO/12", "", "", "", "", "-1", "-1", ""], ["INS-DVL", "IDE_P/DO/13", "", "", "", "", "-1", "-1", ""], ["Multibeam Sonar", "IDE_P/DO/39", "", "", "", "", "-1", "-1", ""], ["SVP, Turbidity, pH", "IDE_P/DO/33", "", "", "", "", "-1", "-1", ""], ["CO2 Sensor", "IDE_P/DO/34", "", "", "", "", "-1", "-1", ""], ["Trim System", "IDE_P/DO/35", "", "", "", "", "-1", "-1", ""], ["Methane_Sensor", "IDE_P/DO/36", "", "", "", "", "-1", "-1", ""], ["VBS", "IDE_P/DO/37", "", "", "", "", "-1", "-1", ""], ["MBS", "IDE_P/DO/39", "", "", "", "", "-1", "-1", ""], ["4K camera S", "IDE_S/DO/0", "", "", "", "", "-1", "-1", ""], ["HD Camera S1", "IDE_S/DO/1", "", "", "", "", "-1", "-1", ""], ["HD Camera S2", "IDE_S/DO/2", "", "", "", "", "-1", "-1", ""], ["HD Camera S3", "IDE_S/DO/3", "", "", "", "", "-1", "-1", ""], ["SD Camera S4", "IDE_S/DO/4", "", "", "", "", "-1", "-1", ""], ["Pan and Tilt S", "IDE_S/DO/5", "", "", "", "", "-1", "-1", ""], ["Laser Light 3", "IDE_S/DO/6", "", "", "", "", "-1", "-1", ""], ["Laser Light 4", "IDE_S/DO/7", "", "", "", "", "-1", "-1", ""], ["LED Light S2", "IDE_S/DO/8", "", "", "", "", "-1", "-1", ""], ["LED Light S3", "IDE_S/DO/9", "", "", "", "", "-1", "-1", ""], ["LED Light S4", "IDE_S/DO/10", "", "", "", "", "-1", "-1", ""], ["Imaging Sonar", "IDE_S/DO/32", "", "", "", "", "-1", "-1", ""], ["Altimeter", "IDE_S/DO/33", "", "", "", "", "-1", "-1", ""], ["Subbottom Profiler", "IDE_S/DO/34", "", "", "", "", "-1", "-1", ""], ["Magnetometer", "IDE_S/DO/35", "", "", "", "", "-1", "-1", ""], ["Conduct & Temp", "IDE_S/DO/36", "", "", "", "", "-1", "-1", ""], ["Dissolved Oxygen", "IDE_S/DO/37", "", "", "", "", "-1", "-1", ""], ["Plume Detector ", "IDE_S/DO/38", "", "", "", "", "-1", "-1", ""], ["Heat Probe Sensor", "IDE_S/DO/39", "", "", "", "", "-1", "-1", ""], ["Thrusters_T1", "", "", "", "", "", "-1", "-1", ""], ["Thrusters _T3", "", "", "", "", "", "-1", "-1", ""], ["Thrusters _T5", "", "", "", "", "", "-1", "-1", ""], ["Thrusters _T7", "", "", "", "", "", "-1", "-1", ""], ["T1Power", "PDE_P/DO/4", "", "", "", "", "-1", "-1", ""], ["T3Power", "PDE_P/DO/5", "", "", "", "", "-1", "-1", ""], ["T5Power", "PDE_P/DO/6", "", "", "", "", "-1", "-1", ""], ["T7Power", "PDE_P/DO/7", "", "", "", "", "-1", "-1", ""], ["BATS_P", "PDE_P/DO/8", "", "", "", "", "-1", "-1", ""], ["OIM RESET _P1", "PDE_P/DO/9", "", "", "", "", "-1", "-1", ""], ["OIM RESET_P2", "PDE_P/DO/10", "", "", "", "", "-1", "-1", ""], ["148 V LED P1", "PDE_P/DO/11", "", "", "", "", "-1", "-1", ""], ["148 V LED P2", "PDE_P/DO/12", "", "", "", "", "-1", "-1", ""], ["148 V LED P3", "PDE_P/DO/13", "", "", "", "", "-1", "-1", ""], ["148 V LED P4", "PDE_P/DO/14", "", "", "", "", "-1", "-1", ""], ["T2-Signal", "PDE_S/DO/0", "", "", "", "", "-1", "-1", ""], ["T4-Signal", "PDE_S/DO/1", "", "", "", "", "-1", "-1", ""], ["T6-Signal", "PDE_S/DO/2", "", "", "", "", "-1", "-1", ""], ["T8-Signal", "PDE_S/DO/3", "", "", "", "", "-1", "-1", ""], ["T2Power", "PDE_S/DO/4", "", "", "", "", "-1", "-1", ""], ["T4Power", "PDE_S/DO/5", "", "", "", "", "-1", "-1", ""], ["T6Power", "PDE_S/DO/6", "", "", "", "", "-1", "-1", ""], ["T8Power", "PDE_S/DO/7", "", "", "", "", "-1", "-1", ""], ["BATS_S", "PDE_S/DO/8", "", "", "", "", "-1", "-1", ""], ["OIM RESET _S1", "PDE_S/DO/9", "", "", "", "", "-1", "-1", ""], ["OIM RESET_S2", "PDE_S/DO/10", "", "", "", "", "-1", "-1", ""], ["148 V LED S1", "PDE_S/DO/11", "", "", "", "", "-1", "-1", ""], ["148 V LED S2", "PDE_S/DO/12", "", "", "", "", "-1", "-1", ""], ["148 V LED S3", "PDE_S/DO/13", "", "", "", "", "-1", "-1", ""], ["148 V LED S4", "PDE_S/DO/14", "", "", "", "", "-1", "-1", ""], ["T1-Signal", "PDE_P/DO/0", "", "", "", "", "-1", "-1", ""], ["T3-Signal", "PDE_P/DO/1", "", "", "", "", "-1", "-1", ""], ["T5-Signal", "PDE_P/DO/2", "", "", "", "", "-1", "-1", ""], ["T7-Signal", "PDE_P/DO/3", "", "", "", "", "-1", "-1", ""], ["Heading", "IDE_P/com1/1", "", "", "", "", "65", "-1", ""], ["Current (A)_P", "TCP/4004/1", "", "", "", "", "44", "-1", ""], ["AUX_P Volt (V)", "TCP/4004/2", "", "", "", "", "43", "-1", ""], ["AUX_P SOC (%)", "TCP/4004/3", "", "", "", "", "46", "-1", ""], ["Roll", "IDE_P/com1/2", "", "", "", "", "63", "-1", ""], ["Pitch", "IDE_P/com1/3", "", "", "", "", "64", "-1", ""], ["Latitude", "IDE_P/com1/4", "", "", "", "", "66", "-1", ""], ["Longitude", "IDE_P/com1/5", "", "", "", "", "67", "-1", ""], ["Depth", "TCP/4003/1", "", "", "", "", "72", "-1", ""], ["Lateral\nSpeed", "IDE_P/com1/7", "", "", "", "", "69", "6", ""], ["Vertical    Speed", "IDE_P/com1/8", "", "", "", "", "70", "7", ""], ["Forward\nSpeed", "IDE_P/com1/9", "", "", "", "", "71", "8", ""], ["T2 Voltage", "PDE_S/com10/2", "", "", "", "", "272", "-1", ""], ["T2 C.Temp", "PDE_S/com10/6", "", "", "", "", "275", "-1", ""], ["T2 Speed", "PDE_S/com10/10", "", "", "", "", "274", "-1", ""], ["T4 Voltage", "PDE_S/com11/2", "", "", "", "", "278", "-1", ""], ["T4 C.Temp", "PDE_S/com11/6", "", "", "", "", "281", "-1", ""], ["T4 Speed", "PDE_S/com11/10", "", "", "", "", "280", "-1", ""], ["T6 Voltage", "PDE_S/com12/2", "", "", "", "", "284", "-1", ""], ["T6 C.Temp", "PDE_S/com12/6", "", "", "", "", "287", "-1", ""], ["T6 Speed", "PDE_S/com12/10", "", "", "", "", "286", "-1", ""], ["T8 Voltage", "PDE_S/com13/2", "", "", "", "", "290", "-1", ""], ["T8 C.Temp", "PDE_S/com13/6", "", "", "", "", "293", "-1", ""], ["T8 Speed", "PDE_S/com13/10", "", "", "", "", "292", "-1", ""], ["AUX_P Current (A)", "TCP/4002/4", "", "", "", "", "43", "35", ""], ["AUX_P Volt (V)", "TCP/4002/11", "", "", "", "", "42", "36", ""], ["AUX_P SOC (%)", "TCP/4002/10", "", "", "", "", "45", "37", ""], ["MB_P Volt (V)", "TCP/4007/2", "", "", "", "", "53", "32", ""], ["MP_P Current (A)", "TCP/4007/1", "", "", "", "", "54", "33", ""], ["MB_P SOC (%)", "TCP/4007/3", "", "", "", "", "56", "34", ""], ["MB_P Temp (deg C)", "TCP/4007/5", "", "", "", "", "57", "-1", ""], ["T1 Voltage", "PDE_P/com10/2", "", "", "", "", "124", "-1", ""], ["T1 Temp", "PDE_P/com10/6", "", "", "", "", "126", "-1", ""], ["T1 Speed", "PDE_P/com10/10", "", "", "", "", "123", "-1", ""], ["T3 Voltage", "PDE_P/com11/2", "", "", "", "", "128", "-1", ""], ["T3  Temp", "PDE_P/com11/6", "", "", "", "", "130", "-1", ""], ["T3 Speed", "PDE_P/com11/10", "", "", "", "", "127", "-1", ""], ["T5 Voltage", "PDE_P/com12/2", "", "", "", "", "132", "-1", ""], ["T5 Temp", "PDE_P/com12/6", "", "", "", "", "134", "-1", ""], ["T5 Speed", "PDE_P/com12/10", "", "", "", "", "131", "-1", ""], ["T7 Voltage", "PDE_P/com13/2", "", "", "", "", "136", "-1", ""], ["T7 Temp", "PDE_P/com13/6", "", "", "", "", "138", "-1", ""], ["T7 Speed", "PDE_P/com13/10", "", "", "", "", "135", "-1", ""], ["BAT CUR", "TCP/4007/1", "", "", "", "", "-1", "-1", ""], ["BAT VOL", "TCP/4007/2", "", "", "", "", "-1", "-1", ""], ["BAT SOC", "TCP/4007/3", "", "", "", "", "-1", "-1", ""], ["BAT TEMP", "TCP/4007/5", "", "", "", "", "-1", "-1", ""], ["Current_1", "TCP/4007/22", "", "", "", "", "163", "-1", ""], ["Voltage_1", "TCP/4007/23", "", "", "", "", "164", "-1", ""], ["ID Cell Max_1", "TCP/4007/24", "", "", "", "", "165", "-1", ""], ["Max Temp_1", "TCP/4007/25", "", "", "", "", "166", "-1", ""], ["ID Cell Min _1 ", "TCP/4007/26", "", "", "", "", "167", "-1", ""], ["Min Temp_1", "TCP/4007/27", "", "", "", "", "168", "-1", ""], ["Temp_1", "TCP/4007/28", "", "", "", "", "169", "-1", ""], ["SOC_1", "TCP/4007/29", "", "", "", "", "170", "-1", ""], ["SOH_1", "TCP/4007/30", "", "", "", "", "171", "-1", ""], ["Current_2", "TCP/4007/37", "", "", "", "", "172", "-1", ""], ["Voltage_2", "TCP/4007/38", "", "", "", "", "173", "-1", ""], ["ID Cell Max_2", "TCP/4007/39", "", "", "", "", "174", "-1", ""], ["Max Temp_2", "TCP/4007/40", "", "", "", "", "175", "-1", ""], ["ID Cell Min _2", "TCP/4007/41", "", "", "", "", "176", "-1", ""], ["Min Temp_2", "TCP/4007/42", "", "", "", "", "177", "-1", ""], ["Temp_2", "TCP/4007/43", "", "", "", "", "178", "-1", ""], ["SOC_2", "TCP/4007/44", "", "", "", "", "179", "-1", ""], ["SOH_2", "TCP/4007/45", "", "", "", "", "180", "-1", ""], ["Current_3", "TCP/4007/52", "", "", "", "", "181", "-1", ""], ["Voltage_3", "TCP/4007/53", "", "", "", "", "182", "-1", ""], ["ID Cell Max_3", "TCP/4007/54", "", "", "", "", "183", "-1", ""], ["Max Temp_3", "TCP/4007/55", "", "", "", "", "184", "-1", ""], ["ID Cell Min _3", "TCP/4007/56", "", "", "", "", "185", "-1", ""], ["Min Temp_3", "TCP/4007/57", "", "", "", "", "186", "-1", ""], ["Temp_3", "TCP/4007/58", "", "", "", "", "187", "-1", ""], ["SOC_3", "TCP/4007/59", "", "", "", "", "188", "-1", ""], ["SOH_3", "TCP/4007/60", "", "", "", "", "189", "-1", ""], ["Current_4", "TCP/4007/67", "", "", "", "", "190", "-1", ""], ["Voltage_4", "TCP/4007/68", "", "", "", "", "191", "-1", ""], ["ID Cell Max_4", "TCP/4007/69", "", "", "", "", "192", "-1", ""], ["Max Temp_4", "TCP/4007/70", "", "", "", "", "193", "-1", ""], ["ID Cell Min _4", "TCP/4007/71", "", "", "", "", "194", "-1", ""], ["Min Temp_4", "TCP/4007/72", "", "", "", "", "195", "-1", ""], ["Temp_4", "TCP/4007/73", "", "", "", "", "196", "-1", ""], ["SOC_4", "TCP/4007/74", "", "", "", "", "197", "-1", ""], ["SOH_4", "TCP/4007/75", "", "", "", "", "198", "-1", ""], ["Current_5", "TCP/4007/82", "", "", "", "", "199", "-1", ""], ["Voltage_5", "TCP/4007/83", "", "", "", "", "200", "-1", ""], ["ID Cell Max_5", "TCP/4007/84", "", "", "", "", "201", "-1", ""], ["Max Temp_5", "TCP/4007/85", "", "", "", "", "202", "-1", ""], ["ID Cell Min _5", "TCP/4007/86", "", "", "", "", "203", "-1", ""], ["Min Temp_5", "TCP/4007/87", "", "", "", "", "204", "-1", ""], ["Temp_5", "TCP/4007/88", "", "", "", "", "205", "-1", ""], ["SOC_5", "TCP/4007/89", "", "", "", "", "206", "-1", ""], ["SOH_5", "TCP/4007/90", "", "", "", "", "207", "-1", ""], ["Altitude", "TCP/4009/1", "", "", "", "", "68", "5", ""], ["S_Heading", "TCP/8110/1", "", "", "", "", "75", "0", ""], ["S_Roll", "TCP/8110/2", "", "", "", "", "73", "1", ""], ["S_Pitch", "TCP/8110/3", "", "", "", "", "74", "2", ""], ["S_Latitude", "TCP/8110/4", "", "", "", "", "76", "3", ""], ["S_Longitude", "TCP/8110/5", "", "", "", "", "77", "4", ""], ["S_Depth", "TCP/4010/1", "", "", "", "", "78", "9", ""], ["T1 ctrl", " PDE_P/com10/9", "", "", "", "", "155", "-1", ""], ["T3 ctrl", " PDE_P/com11/9", "", "", "", "", "156", "-1", ""], ["T5 ctrl", " PDE_P/com12/9", "", "", "", "", "157", "-1", ""], ["T7 ctrl ", " PDE_P/com13/9", "", "", "", "", "158", "-1", ""], ["T2 ctrl ", " PDE_S/com10/9", "", "", "", "", "159", "-1", ""], ["T4 ctrl", " PDE_S/com11/9", "", "", "", "", "160", "-1", ""], ["T6 ctrl", " PDE_S/com12/9", "", "", "", "", "161", "-1", ""], ["T8 ctrl", " PDE_S/com13/9", "", "", "", "", "162", "-1", ""], ["CO2_s ", "", "", "", "", "", "92", "10", ""], ["Oxygen_S", "", "", "", "", "", "93", "11", ""], ["Presssure in mbar_S", "", "", "", "", "", "94", "12", ""], ["Temp in Deg C_S", "", "", "", "", "", "95", "13", ""], ["Humidity_S in %", "", "", "", "", "", "96", "14", ""], ["CO2_P ", "", "", "", "", "", "102", "15", ""], ["Oxygen_P", "", "", "", "", "", "103", "16", ""], ["Presssure in mbar_P", "", "", "", "", "", "104", "17", ""], ["Temp in Deg C_P", "", "", "", "", "", "105", "18", ""], ["Humidity_P in %", "", "", "", "", "", "106", "19", ""], ["MB_S Volt (V)", "", "", "", "", "", "58", "20", ""], ["MB_S Current (A)", "", "", "", "", "", "59", "21", ""], ["MB_S SOC (%)", "", "", "", "", "", "61", "22", ""], ["AUX_S Volt (V)", "", "", "", "", "", "48", "23", ""], ["AUX_S Current (A)", "", "", "", "", "", "49", "24", ""], ["AUX_S SOC (%)", "", "", "", "", "", "51", "25", ""], ["PDE_S IR (Kohm)", "PDE_S/com20/1", "", "", "", "", "267", "30", ""], ["IDE_S IR  (Kohm)", "IDE_S/com13/1", "", "", "", "", "271", "31", ""], ["PDE_P IR (Kohm)", "", "", "", "", "", "-1", "42", ""], ["IDE_P IR (kohm)", "", "", "", "", "", "6", "43", ""], ["S_ALGSTS_M", "TCP/8110/16", "", "", "", "", "-1", "-1", ""], ["S_ALGSTS_L", "TCP/8110/17", "", "", "", "", "-1", "-1", ""], ["S_STATUS_M", "TCP/8110/18", "", "", "", "", "-1", "-1", ""], ["S_STATUS_L", "TCP/8110/19", "", "", "", "", "-1", "-1", ""], ["S_HTSTATUS", "TCP/8110/20", "", "", "", "", "-1", "-1", ""], ["Dissolved O2", "IDE_S/DO/12", "", "", "", "", "-1", "-1", ""], ["Disolved Oxygen", "TCP/4112/5", "", "", "", "", "262", "-1", ""], ["Subea Temp_2", "TCP/4112/11", "", "", "", "", "263", "-1", ""], ["Altitude", "TCP/4113/1", "", "", "", "", "261", "-1", ""], ["T2 W. Temp ", "PDE_S/com10/7", "", "", "", "", "277", "-1", ""], ["T4 W. Temp ", "PDE_S/com11/7", "", "", "", "", "283", "-1", ""], ["T6 W. Temp ", "PDE_S/com12/7", "", "", "", "", "289", "-1", ""], ["T8 W. Temp ", "PDE_S/com13/7", "", "", "", "", "295", "-1", ""], ["T2 HS.Temp", "PDE_S/com10/5", "", "", "", "", "276", "-1", ""], ["T4 HS.Temp", "PDE_S/com11/5", "", "", "", "", "282", "-1", ""], ["T6 HS.Temp ", "PDE_S/com12/5", "", "", "", "", "288", "-1", ""], ["T8 HS.Temp", "PDE_S/com13/5", "", "", "", "", "294", "-1", ""]]
  (unwired) string[] ["PS_P", "IDE_P", "PS_S", "PDE_S", "PDE_P", "IDE_S"] ("Addresses")
  w48 = string[] ["Imaging", "Sensors", "Logging", "STATUS", "MCC", "50 Kwh"]  # Co-Pilot Tab
  w49 = string[] ["Main", "HSSS ", "Ballast", "Propulsion", "Power "]  # Pilot Tab
  # "IDE_S/DO/1\n\nDissolved o2"
  # "Wago plc"
  # "MCC"
  # "T3 ctrl             PDE_P/com10/9    T3 ctrl             PDE_P/com11/9\nT5 ctrl             PDE_P/com12/9\nT7 ctrl              PDE_P/com13/9\nT2 ctrl               PDE_S/com10/9\nT4 ctrl                PDE_S/com11/9\nT6 ctrl               PDE_S/com12/9\nT8 ctrl                PDE_S/com13/9"
  # "T2 ctrl"
  # "PDE_S/com10/8"
  # "6 Logging Index"
  # "0 Control Name"
  # "1 Target, channel type and Index"
  # "2 Multiplication Factor"
  # "5 DI Channel"
  # "4 DO channel"
  # "3 Threshold Value"
  # "INS DVL, 4003\n\nHEADING_1\nROLL\nPITCH\nLatitude\nLongitude\nAltitude\nEast speed\nNorth speed\nUP speed\nDepth\nLat GPS\nLong GPS\nAltitude GPS\nSURGE\nSWAY\nHEAVE"
  # "old table"
  # "LS02"
  # "PDE_S/AI/11"
  # "129\n145\n133\n149\n141\n137\n153\n125"
  # "T3  Current\nT4 Current\nT5 Current\nT6 Current\nT2 Current\nT7 Current\nT8 Current\nT1 Current"
  # "PDE_P/AI/5\nPDE_P/AI/6\nPDE_S/AI/6\nPDE_P/AI/7\nPDE_S/AI/7\nPDE_S/AI/5\nPDE_P/AI/8\nPDE_S/AI/8"
  # "T1 Current\nPDE_P/AI/5\n7.5"
  # "LOGGING INDEX 47 not mapped AUX_P Temp (deg C)\n                               50  not mapped AUX _s power\n                               52   AUX _S Temp\n                               55 MB_P power\n                               60 MB_S Power\n                               62 MB_S Temp\n                               79 depth sensor primary \n                               80 depth sensor secondary\n                               81 ALTITUDE 2\n                               97 - 122 NOT MAPPED BALLAST NOT MAPPED"
  # "IDE_S/DO/1\n\nDissolved o2"
  # "Wago plc"
  # "MCC"
  # "T3 ctrl             PDE_P/com10/9    T3 ctrl             PDE_P/com11/9\nT5 ctrl             PDE_P/com12/9\nT7 ctrl              PDE_P/com13/9\nT2 ctrl               PDE_S/com10/9\nT4 ctrl                PDE_S/com11/9\nT6 ctrl               PDE_S/com12/9\nT8 ctrl                PDE_S/com13/9"
  # "T2 ctrl"
  # "PDE_S/com10/8"
  # "6 Logging Index"
  # "Battery5\n81 Power\n82Current\n83 Pack Voltage\n84ID cell max\n85Max temperature\n86 ID Cell min\n87 Min temperature\n88 Temperature\n89 SOC\n90 SOH\n91 State Bat\n92Flags Bat\n93Fault Code\n94 Level Faults\n95Warnings"
  # "Battery4\n66 Power\n67Current\n68 Pack Voltage\n69ID cell max\n70Max temperature\n71 ID Cell min\n72 Min temperature\n73 Temperature\n74 SOC\n75 SOH\n76 State Bat\n77Flags Bat\n78 Fault Code\n79 Level Faults\n80Warnings"
  # "Global Data\n01 Battery Current\n02 Battery Voltage\n03 SOC\n04 SOH\n05 Mean Temperature\n06 Status Faults\n07 Status Warning\n08 Status battery\n\nSummary 10 kW modules\n09 Battery ID\n10 Max temperature\n11 Pack Max voltage\n12 battrey ID Voltgae\n13 Battery ID Min Voltage\n14 Pack Min Voltage\n15 Battery ID min\n16 ID cell Min\n17 Min Cell Voltage\n18 Battery ID Max\n19 ID cell Max\n20 Max cell voltage\n\nEach 10 kW Batteries                                                        \nBattery1\n21 Power\n22 Current\n23 Pack Voltage\n24 ID cell max\n25 Max temperature\n26 ID Cell min\n27 Min temperature\n28 Temperature\n29 SOC\n30 SOH\n31 State Bat\n32 Flags Bat\n33 Fault Code\n34 Level Faults\n35 Warnings\n\nBattery2\n36 Power\n37 Current\n38 Pack Voltage\n39 ID cell max\n40 Max temperature\n41 ID Cell min\n42 Min temperature\n43 Temperature\n44 SOC\n45 SOH\n46 State Bat\n47 Flags Bat\n48 Fault Code\n49 Level Faults\n50 Warnings\n\n\n\nBattery3\n51 Power\n52Current\n53 Pack Voltage\n54 ID cell max\n55Max temperature\n56 ID Cell min\n57 Min temperature\n58 Temperature\n59 SOC\n60 SOH\n61 State Bat\n62 Flags Bat\n63 Fault Code\n64 Level Faults\n65Warnings"
  # "Global Data\n01 Battery Current\n02 Battery Voltage\n03 SOC\n04 SOH\n05 Mean Temperature\n06 Status Faults\n07 Status Warning\n08 Status battery\n\nSummary 10 kW modules\n09 Battery ID\n10 Max temperature\n11 Pack Max voltage\n12 battrey ID Voltgae\n13 Battery ID Min Voltage\n14 Pack Min Voltage\n15 Battery ID min\n16 ID cell Min\n17 Min Cell Voltage\n18 Battery ID Max\n19 ID cell Max\n20 Max cell voltage\n\nEach 10 kW Batteries\n21 Power\n22 Current\n23 Pack Voltage\n24 ID cell max\n25 Max temperature\n26 ID Cell min\n27 Min temperature\n28 Temperature\n29 SOC\n30 SOH\n31 State Bat\n32 Flags Bat\n33 Fault Code\n34 Level Faults\n35 Warnings"
  # "0 Control Name"
  # "1 Target, channel type and Index"
  # "2 Multiplication Factor"
  # "5 DI Channel"
  # "4 DO channel"
  # "3 Threshold Value"
  # "4002 - 10KW Batery\n\n01 S No\n02 Date\n03 Time\n\nContext Data\n\n04  Level faults\n05  No of on/off cycles\n06  Time since power came on\n07  Source current (mA)\n08  Load Current (mA)\n09  State of Certain i/p and o/p\n10  CCL (%)\n11  DCL (%)\n12  Relay State machine state\n13  SOC (%)\n14  Pack Total Voltage (V)\n15  No of a bank missing\n16  No of missing cells\n17  No of a missing cell\n18  Min. Cell Voltage (V)\n19  No of Cell with lowest Voltge\n20  Avg Cell Voltage (V)\n21  Max. Cell Voltage (V)\n22  No of cell with the highest voltage\n23  Min. Cell Board Temperature (°C)\n24  No of Cell Board with Lowest Temp\n25  Avg. Cell Board Temperature (°C)\n26  Max. Cell Board Temperature (°C)\n27  No of cell Cell Board with Highest Temp\n28  No of Loads that are on\n29  Cell Voltage Above which we turn on its load \n\nAuxilary Data\n\n30 State\n31 Level fault flags\n32 Total energy in of battery (kWH)\n33 Total energy out of battery (kWH)\n34 DOD (Ah)\n35 Capacity [Ah] \n36 SOH (%)\n37 Pack Resistance (µOhm)\n38 Min. Cell Resistance (µOhm)\n39 Number of cell with minimum resistance\n40 Avg. Cell Resistance (µOhm)  \n41 Max. Cell Resistance (µOhm) \n42 Number of cell with maximum resistance\n43 Number of cells seen\n44 Power (W)"
  # "INS DVL, 4003\n\nHEADING_1\nROLL\nPITCH\nLatitude\nLongitude\nAltitude\nEast speed\nNorth speed\nUP speed\nDepth\nLat GPS\nLong GPS\nAltitude GPS\nSURGE\nSWAY\nHEAVE"
  n1 = call "Host - Launch Target VIs (SubVI).vi"("error in"="error in", "IP"=w2) -> ("error out"=w40:errorcluster, "VI Ref"=w51:refnum<vi>[], "Channel Data"=w30:T17, "DO"=w53:T7[], "DI"=w31:T7[])  [unwired: 5 in]
  n2 = property class="TabCtl"(reference="Tab Reference") -> ("Pages"=w50:refnum<vi>[])  [unwired: 1 in, 2 out]
  n3 = call "Host - extract control Ref.vi"("Co-Pilot Tab"=w48, "Pilot Tab"=w49, "Pages"=w50) -> ("All Controls"=w44:refnum<vi>[], "Co-Pilot Controls"=w33:refnum<vi>[], "Pilot Controls"=w47:refnum<vi>[])  [unwired: 5 in, 1 out]
  n4 = for {
    tunnel: w44 -> [w56] mode=indexing
    tunnel: [w55] -> w45 mode=indexing
    n5 = property class="Ctl"(reference=w56) -> ("Label.Text"=w55:string)  [unwired: 1 in, 2 out]
  }
  n6 = call "Host - Configure Default Data.vi"("DO"=w53, "DI"=w31, "Source"=w2) -> ("DO Data"=w26:cluster{"Names":string[], "Data":bool[]}[], "DI Data"=w29:cluster{bool[]}[])  [unwired: 7 in]
  n7 = call "Host - Sort Controls.vi"("Controls"=w47) -> ("Array"=→"Array":u32[], "Names"=w6:string[], "Sorted Ref"=w7:refnum<vi>[])  [unwired: 8 in]
  "Names" <- w6
  "output array" <- w7
  n8 = call "Host - Sort Controls.vi"("Controls"=w33) -> ("Names"=w4:string[], "Sorted Ref"=w5:refnum<vi>[])  [unwired: 8 in, 1 out]
  "Names 3" <- w4
  n9 = Index Array(array=w1, index (col)=0 ("disabled index (col)")) -> (element=→"Control names":string[])  [unwired: 1 in]
  n10 = Bundle(w45, "All Controls"=w44) -> (w46:cluster{string[], "All Controls":refnum<vi>[]})  [unwired: 1 in]
  n11 = Obtain Queue(max queue size (-1, unlimited)=5000, name (unnamed)="TCP-Serial", element data type=string[] [], error in (no error)=w40) -> (queue out=w18:refnum<queue>, error out=w35:errorcluster)  [unwired: 1 in, 1 out]
  n12 = call "Host - Launch TCP Serial VIs (SubVI).vi"() -> ("TCP Serial Data"=w28:string[][], "TCP Serial Ref"=w39:refnum<vi>[])  [unwired: 10 in]
  n13 = Initialize Array(w15, 43 ("dimension size")) -> (w16:sgl[])
  n14 = call "Notifier get and set.vi"("Operation"=enum16{"Init", "Get", "Set"}."Init") -> ("notifier out"=w14:refnum<notifier>)  [unwired: 9 in, 1 out]
  n15 = Initialize Array(w15, 296 ("dimension size")) -> (w19:sgl[])
  n16 = call "Wago notifier.vi"("Operation"=enum16{"Init", "Get", "Set"}."Init") -> ("notifier out"=w12:refnum<notifier>)  [unwired: 9 in, 1 out]
  n17 = call "Host - Seggregate DO names.vi"("Co-Pilot Control Names"=w1, "Pilot Control Names"=w4, "GUI Data"=w6) -> ("Co-Pilot DO"=w23:cluster{"Data":i32[]}[], "Pilot DO"=w24:cluster{"Data":i32[]}[])  [unwired: 7 in]
  n18 = call "Host - Alarm Init (SubVI).vi"("GUI Data in"=w1) -> ("Alarm Index"=w36:T18)  [unwired: 10 in]
  n19 = Initialize Array(sgl 0.0 ("element"), 65 ("dimension size")) -> (w8:sgl[])
  n20 = Bundle By Name(cluster=T2 {"VI References"=[], "Addresses"=[], "Pilot"=FALSE, "DO Data"=[], "Access Restricted?"=FALSE, "Pilot Control References"=[], "CoPilot Control References"=[], "cRIO Config"=[], "datalog Q"=refnum, "PS_P"={"AI"=[], "DI"=[], "DO"=[], "Serial"=[], "CPU"={"Total Load"=[], "Interrupt Load"=[], "Total Physical"=0.0, "Free Physical"=0.0, "Primary Disk Capacity"=0.0, "Primary Disk Free"=0.0}, "Stop"=FALSE, "DO Channel"=[]}, "PS_S"={"AI"=[], "DI"=[], "DO"=[], "Serial"=[], "CPU"={"Total Load"=[], "Interrupt Load"=[], "Total Physical"=0.0, "Free Physical"=0.0, "Primary Disk Capacity"=0.0, "Primary Disk Free"=0.0}, "Stop"=FALSE, "DO Channel"=[]}, "IDE_P"={"AI"=[], "DI"=[], "DO"=[], "Serial"=[], "CPU"={"Total Load"=[], "Interrupt Load"=[], "Total Physical"=0.0, "Free Physical"=0.0, "Primary Disk Capacity"=0.0, "Primary Disk Free"=0.0}, "Stop"=FALSE, "DO Channel"=[]}, "IDE_S"={"AI"=[], "DI"=[], "DO"=[], "Serial"=[], "CPU"={"Total Load"=[], "Interrupt Load"=[], "Total Physical"=0.0, "Free Physical"=0.0, "Primary Disk Capacity"=0.0, "Primary Disk Free"=0.0}, "Stop"=FALSE, "DO Channel"=[]}, "PDE_P"={"AI"=[], "DI"=[], "DO"=[], "Serial"=[], "CPU"={"Total Load"=[], "Interrupt Load"=[], "Total Physical"=0.0, "Free Physical"=0.0, "Primary Disk Capacity"=0.0, "Primary Disk Free"=0.0}, "Stop"=FALSE, "DO Channel"=[]}, "PDE_S"={"AI"=[], "DI"=[], "DO"=[], "Serial"=[], "CPU"={"Total Load"=[], "Interrupt Load"=[], "Total Physical"=0.0, "Free Physical"=0.0, "Primary Disk Capacity"=0.0, "Primary Disk Free"=0.0}, "Stop"=FALSE, "DO Channel"=[]}, "GUI References"={"Control Names"=[], "Control References"=[]}, "GUI Data"=[], "TCP - Serial"=[], "TCP-Serial Q"=refnum, "TCP Serial Ref"=[], "Data Sets"=[], "Last Data"=[], "Alarm Data"=[], "DI Data"=[], "Ack Data"=[], "Buzzer Data"=[], "Pilot DO"=[], "Co-Pilot DO"=[], "System Down?"=FALSE, "Log Data"=[], "Update Array"=[], "MCC Data Log"=[], "MCC Data Not"=refnum, "Thruster control"=[refnum, refnum, refnum, refnum, refnum, refnum, refnum, refnum, refnum], "waga notifier out"=refnum, "Wago  log"=[], "Thruster Cont"=[0.0, 0.0, 0.0, 0.0, 0.0, 0.0, 0.0, 0.0, 0.0, 0.0, 0.0], "Cam Cont"=[FALSE, FALSE, FALSE, FALSE, FALSE, TRUE], "PDE_P TH Cont"={"COM 10"=0.0, "COM 11"=0.0, "COM 12"=0.0, "COM 13"=0.0}, "PDE_S TH Cont"={"COM 10"=0.0, "COM 11"=0.0, "COM 12"=0.0, "COM 13"=0.0}} ("Data Cluster 2"), "Pilot"="Pilot", "DI Data"=w29, "DO Data"=w26, "Addresses"=w2, "VI References"=w51, "cRIO Config"=w30, "Pilot Control References"=w7, "CoPilot Control References"=w5, "GUI References"=w46, "TCP-Serial Q"=w18, "TCP Serial Ref"=w39, "TCP - Serial"=w28, "GUI Data"=w1, "Alarm Data"=w36, "Data Sets"=dbl[][] [], "Pilot DO"=w24, "Co-Pilot DO"=w23, "Log Data"=w19, "MCC Data Log"=w16, "MCC Data Not"=w14, "waga notifier out"=w12, "Wago  log"=w8) -> (→"Data Cluster":T2)
  n21 = call "Host - Update Data Cluster.vi"("Operation"=enum16{"Init", "Get", "Set"}."Init", "error in"=w35) -> ("error out"=→"error out":errorcluster)  [unwired: 8 in, 1 out]
